vi "Send Stop.vi"(9 "sync in":errorcluster) -> (2 "channel out":T1)   [LabVIEW 2019, in "Cmd-Data Event Messages.lvlib"]
doc: "Sends the message of command STOP with an empty data variant to the channel connected to this VI. This VI executes normally even if there is an error at sync in."
uses:
  Cmd-Data Event Messages.lvlib
  cmd-data event messenger/source/Cmd-Data Event Messenger.lvlib
  cmd-data event messenger/source/))Channel.ctl
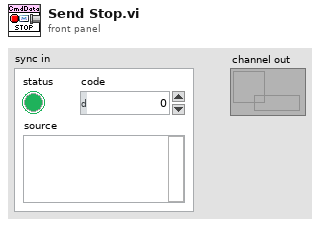
[diagram p1: front panel]
types:
  T1 = typedef "Cmd-Data Event Messenger.lvlib/))Channel.ctl" = refnum<queue>
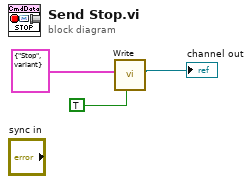
[diagram p0: block diagram]
diagram:
  n1 = call "Write.vi"("high priority? (F)"=TRUE, "element"=cluster{"cmd":string, "data":variant} {"cmd"="Stop", "data"=variant} ("message")) -> ("channel out"=→"channel out":T1)  [unwired: 8 in, 1 out]
